vi "SVX Combine Filtered and Unfiltered Plots.vi"(8 "error in (no error)":errorcluster, 10 "unfiltered plot":T1(array[cluster]), 11 "filtered plot":T1(array[cluster])) -> (0 "error out":errorcluster, 3 "combined plot":T1(array[cluster]))   [LabVIEW 2017, in "SoundVib_MCMDisplay.lvlib"]
doc: "Combines filtered and unfiltered orbit plots or timebase plots into a single plot. Use this VI to see the relationship between the unfiltered signal and the signal filtered by significant orders."
uses:
  <vilib>/addons/Sound and Vibration/Order Analysis/Data Presentation/SoundVib_MCMDisplay.lvlib
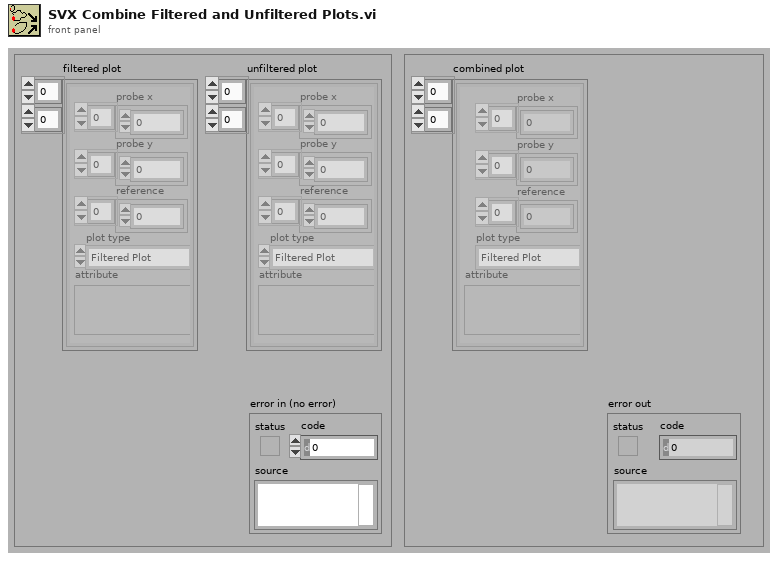
[diagram p1: front panel]
types:
  T1 = cluster{"probe x":dbl[], "probe y":dbl[], "reference":dbl[], "plot type":enum16{"Filtered Plot", "Unfiltered Plot"}, "attribute":variant}[][]
  T2 = cluster{"probe x":dbl[], "probe y":dbl[], "reference":dbl[], "plot type":enum16{"Filtered Plot", "Unfiltered Plot"}, "attribute":variant}[]
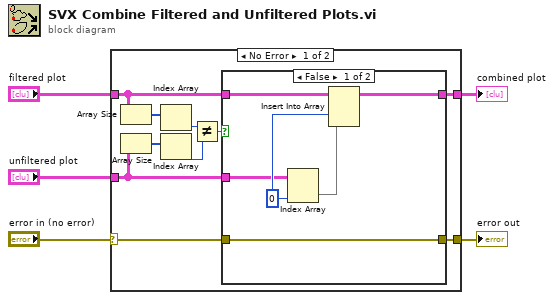
[diagram p0: block diagram]
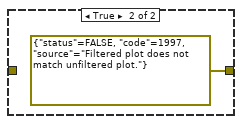
[diagram p2: hidden frame]
diagram:
  n1 = case shown="No Error" "error in (no error)" {
    selector: "error in (no error)" -> [w6 w23]
    tunnel: "unfiltered plot" -> [w11 _]
    tunnel: [w15 _] -> w4
    tunnel: "filtered plot" -> [w14 _]
    tunnel: [w7 w23] -> w1
    frame No Error {
      n2 = Array Size(array=w14) -> (size(s)=w13:i32[])
      n3 = Array Size(array=w11) -> (size(s)=w12:i32[])
      n4 = Index Array(array=w13) -> (element=w10:i32)  [unwired: 1 in]
      n5 = Index Array(array=w12) -> (element=w9:i32)  [unwired: 1 in]
      n6 = Not Equal?(x=w10, y=w9) -> (x != y?=w8:bool)
      n7 = case shown="False" w8 {
        tunnel: [w21 _] -> w15
        tunnel: w14 -> [w18 _]
        tunnel: w11 -> [w17 _]
        tunnel: [w16 errorcluster {"status"=FALSE, "code"=1997, "source"="Filtered plot does not match unfiltered plot."} ("error IO")] -> w7
        tunnel: w6 -> [w16 _]
        frame False {
          w19 = 0 ("index (row)")
          n8 = Index Array(array=w17, index (col)=w19) -> (element=w20:T2)  [unwired: 1 in]
          n9 = Insert Into Array(array=w18, index (col)=w19, new element=w20) -> (w21:T1)  [unwired: 1 in]
        }
        frame True {
        }
      }
    }
    frame Error {
    }
  }
  "combined plot" <- w4
  "error out" <- w1
